vi "MeasurementServer_Stop.vi"(0 "Server Information":T2, 1 "Event Registration Refnum":refnum<event-registration>, 3 "error in (no error)":errorcluster) -> (10 "error out":errorcluster)   [LabVIEW 2019, in "labview-grpc-measurement-server.lvlib"]
uses:
  labview-grpc-measurement-server.lvlib
  MeasurementServer_InvokeEventData.ctl
  MeasurementServer_gRPCid.ctl
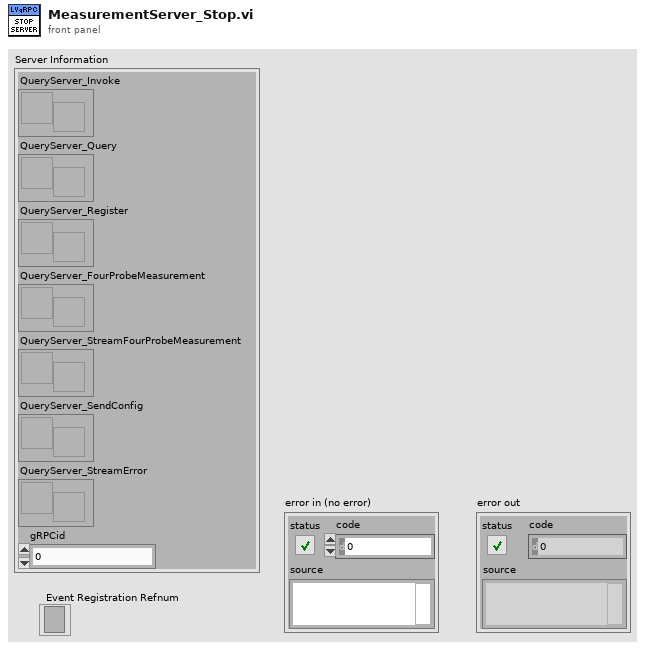
[diagram p1: front panel]
types:
  T1 = typedef "labview-grpc-measurement-server.lvlib/MeasurementServer_gRPCid.ctl" = u64
  T2 = cluster{"QueryServer_Invoke":refnum<user-event>, "QueryServer_Query":refnum<user-event>, "QueryServer_Register":refnum<user-event>, "QueryServer_FourProbeMeasurement":refnum<user-event>, "QueryServer_StreamFourProbeMeasurement":refnum<user-event>, "QueryServer_SendConfig":refnum<user-event>, "QueryServer_StreamError":refnum<user-event>, "gRPCid":T1}
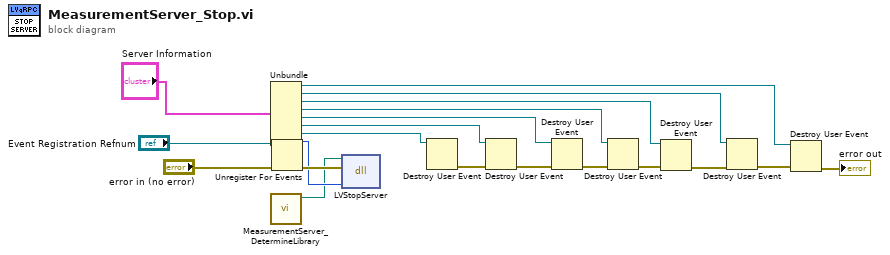
[diagram p0: block diagram]
diagram:
  n1 = Unbundle("Server Information") -> ("QueryServer_Invoke"=w13:refnum<user-event>, "QueryServer_Query"=w14:refnum<user-event>, "QueryServer_Register"=w15:refnum<user-event>, "QueryServer_FourProbeMeasurement"=w11:refnum<user-event>, "QueryServer_StreamFourProbeMeasurement"=w9:refnum<user-event>, "QueryServer_SendConfig"=w7:refnum<user-event>, "QueryServer_StreamError"=w2:refnum<user-event>, "gRPCid"=w4:T1)
  n2 = call "MeasurementServer_DetermineLibrary.vi"() -> ("path out"=w1:path)  [unwired: 11 in]
  n3 = Unregister For Events(event registration refnum="Event Registration Refnum", error in="error in (no error)") -> (error out=w20:errorcluster)
  n4 = dll-call lib="C:/Users/chericks/Desktop/LabVIEW-grpc-measurement-server/build/Debug/labview_measurement_server.dll" fn="LVStopServer"(path in=w1, error in=w20, "server"=w4) -> ()  [unwired: 3 in, 2 out]
  n5 = Destroy User Event(user event=w2) -> (error out=w3:errorcluster)  [unwired: 1 in]
  n6 = Destroy User Event(user event=w7, error in=w3) -> (error out=w8:errorcluster)
  n7 = Destroy User Event(user event=w9, error in=w8) -> (error out=w10:errorcluster)
  n8 = Destroy User Event(user event=w11, error in=w10) -> (error out=w12:errorcluster)
  n9 = Destroy User Event(user event=w15, error in=w12) -> (error out=w18:errorcluster)
  n10 = Destroy User Event(user event=w14, error in=w18) -> (error out=w17:errorcluster)
  n11 = Destroy User Event(user event=w13, error in=w17) -> (error out=→"error out":errorcluster)
